vi "Config.vi"() -> ()   [LabVIEW 2020]
uses:
  Global_Variable/Global.vi
  Global_Variable/A180648.vi
  <vilib>/Utility/config.llb/NI_LVConfig.lvlib
  Libraries/S7/S7.lvlib
panel:
  in  "试验项目":T1
  in  "产品型号":string(combo)
  in  "删除":bool
  in  "确定":bool
  in  "添加":bool
  in  "退出":bool
  in  "更新":bool
  in  "选项卡控件":enum32{"产品参数", "通信参数", "系统参数"}(tab)
  in  "产品参数选项卡":T2(tab)
  in  "输入轴花键参数":string[][](table)=[[""], ["°/s"], ["°"], ["Nm"]]
  in  "输入轴移载参数":string[][](table)=[["mm"], ["mm/s"], ["mm"], ["mm/s"]]
  in  "工装参数":string[][](table)=[["mm"], ["mm/s"]]
  in  "空载判定参数":string[][](table)=[["Nm", "", ""], ["Nm", "", ""], ["Nm", "", ""], ["Nm", "", ""], ["Nm", "", ""], ["Nm", "", ""], ["Nm", "", ""], ["Nm", "", ""], ["Nm", "", ""], ["Nm", "", ""]]
  in  "空载试验参数":string[][](table)=[[""], ["°/s"], ["°"], ["Nm"]]
  in  "功能判定参数":string[][](table)=[["Nm"], ["Nm"], ["Nm"], ["Nm"], ["Nm"], ["Nm"], ["Nm"], ["Nm"], ["Nm"]]
  in  "功能试验参数":string[][](table)=[["°/s"], ["°"], ["Nm"], ["Nm"]]
  in  "车速选项卡":T3(tab)
  in  "力特性试验参数":string[][](table)=[["°/s"], ["Nm"], ["RPM"], ["Km/h"]]
  in  "传感器特性判定参数":string[][](table)=[["V", "", ""], ["V", "", ""], ["V", "", ""], ["V", "", ""], ["V", "", ""], ["V", "", ""], ["V", "", ""], ["V", "", ""], ["V", "", ""], ["V", "", ""], ["V", "", ""], ["V", "", ""], ["V", "", ""], ["V", "", ""]]
  in  "力特性判定参数 0":string[][](table)=[["Nm", "", ""], ["%", "", ""], ["Nm", "", ""], ["Nm", "", ""], ["Nm", "", ""], ["Nm", "", ""], ["Nm", "", ""], ["Nm", "", ""], ["Nm", "", ""], ["Nm", "", ""], ["Nm", "", ""], ["Nm", "", ""], ["Nm", "", ""], ["Nm", "", ""], ["Nm", "", ""], ["Nm", "", ""], ["Nm", "", ""], ["Nm", "", ""], ["Nm", "", ""], ["Nm", "", ""], ["Nm", "", ""], ["Nm", "", ""], ["Nm", "", ""], ["Nm", "", ""], ["Nm", "", ""], ["Nm", "", ""], ["Nm", "", ""]]
  in  "电流特性判定参数 0":string[][](table)=[["Nm", "", ""], ["%", "", ""], ["A", "", ""], ["A", "", ""], ["Nm", "", ""], ["Nm", "", ""], ["Nm", "", ""], ["Nm", "", ""], ["Nm", "", ""], ["Nm", "", ""], ["Nm", "", ""], ["Nm", "", ""], ["Nm", "", ""], ["Nm", "", ""], ["Nm", "", ""], ["Nm", "", ""], ["Nm", "", ""], ["Nm", "", ""], ["Nm", "", ""], ["Nm", "", ""], ["Nm", "", ""], ["Nm", "", ""], ["Nm", "", ""], ["Nm", "", ""], ["Nm", "", ""], ["Nm", "", ""], ["Nm", "", ""], ["Nm", "", ""]]
  in  "电流特性判定参数 1":string[][](table)=[["Nm", "", ""], ["%", "", ""], ["A", "", ""], ["A", "", ""], ["Nm", "", ""], ["Nm", "", ""], ["Nm", "", ""], ["Nm", "", ""], ["Nm", "", ""], ["Nm", "", ""], ["Nm", "", ""], ["Nm", "", ""], ["Nm", "", ""], ["Nm", "", ""], ["Nm", "", ""], ["Nm", "", ""], ["Nm", "", ""], ["Nm", "", ""], ["Nm", "", ""], ["Nm", "", ""], ["Nm", "", ""], ["Nm", "", ""], ["Nm", "", ""], ["Nm", "", ""], ["Nm", "", ""], ["Nm", "", ""], ["Nm", "", ""], ["Nm", "", ""]]
  in  "力特性判定参数 1":string[][](table)=[["Nm", "", ""], ["%", "", ""], ["Nm", "", ""], ["Nm", "", ""], ["Nm", "", ""], ["Nm", "", ""], ["Nm", "", ""], ["Nm", "", ""], ["Nm", "", ""], ["Nm", "", ""], ["Nm", "", ""], ["Nm", "", ""], ["Nm", "", ""], ["Nm", "", ""], ["Nm", "", ""], ["Nm", "", ""], ["Nm", "", ""], ["Nm", "", ""], ["Nm", "", ""], ["Nm", "", ""], ["Nm", "", ""], ["Nm", "", ""], ["Nm", "", ""], ["Nm", "", ""], ["Nm", "", ""], ["Nm", "", ""], ["Nm", "", ""]]
  in  "力特性判定参数 2":string[][](table)=[["Nm", "", ""], ["%", "", ""], ["Nm", "", ""], ["Nm", "", ""], ["Nm", "", ""], ["Nm", "", ""], ["Nm", "", ""], ["Nm", "", ""], ["Nm", "", ""], ["Nm", "", ""], ["Nm", "", ""], ["Nm", "", ""], ["Nm", "", ""], ["Nm", "", ""], ["Nm", "", ""], ["Nm", "", ""], ["Nm", "", ""], ["Nm", "", ""], ["Nm", "", ""], ["Nm", "", ""], ["Nm", "", ""], ["Nm", "", ""], ["Nm", "", ""], ["Nm", "", ""], ["Nm", "", ""], ["Nm", "", ""], ["Nm", "", ""]]
  in  "电流特性判定参数 2":string[][](table)=[["Nm", "", ""], ["%", "", ""], ["A", "", ""], ["A", "", ""], ["Nm", "", ""], ["Nm", "", ""], ["Nm", "", ""], ["Nm", "", ""], ["Nm", "", ""], ["Nm", "", ""], ["Nm", "", ""], ["Nm", "", ""], ["Nm", "", ""], ["Nm", "", ""], ["Nm", "", ""], ["Nm", "", ""], ["Nm", "", ""], ["Nm", "", ""], ["Nm", "", ""], ["Nm", "", ""], ["Nm", "", ""], ["Nm", "", ""], ["Nm", "", ""], ["Nm", "", ""], ["Nm", "", ""], ["Nm", "", ""], ["Nm", "", ""], ["Nm", "", ""]]
  in  "力特性判定参数 3":string[][](table)=[["Nm", "", ""], ["%", "", ""], ["Nm", "", ""], ["Nm", "", ""], ["Nm", "", ""], ["Nm", "", ""], ["Nm", "", ""], ["Nm", "", ""], ["Nm", "", ""], ["Nm", "", ""], ["Nm", "", ""], ["Nm", "", ""], ["Nm", "", ""], ["Nm", "", ""], ["Nm", "", ""], ["Nm", "", ""], ["Nm", "", ""], ["Nm", "", ""], ["Nm", "", ""], ["Nm", "", ""], ["Nm", "", ""], ["Nm", "", ""], ["Nm", "", ""], ["Nm", "", ""], ["Nm", "", ""], ["Nm", "", ""], ["Nm", "", ""]]
  in  "电流特性判定参数 3":string[][](table)=[["Nm", "", ""], ["%", "", ""], ["A", "", ""], ["A", "", ""], ["Nm", "", ""], ["Nm", "", ""], ["Nm", "", ""], ["Nm", "", ""], ["Nm", "", ""], ["Nm", "", ""], ["Nm", "", ""], ["Nm", "", ""], ["Nm", "", ""], ["Nm", "", ""], ["Nm", "", ""], ["Nm", "", ""], ["Nm", "", ""], ["Nm", "", ""], ["Nm", "", ""], ["Nm", "", ""], ["Nm", "", ""], ["Nm", "", ""], ["Nm", "", ""], ["Nm", "", ""], ["Nm", "", ""], ["Nm", "", ""], ["Nm", "", ""], ["Nm", "", ""]]
  in  "电流特性判定参数 4":string[][](table)=[["Nm", "", ""], ["%", "", ""], ["A", "", ""], ["A", "", ""], ["Nm", "", ""], ["Nm", "", ""], ["Nm", "", ""], ["Nm", "", ""], ["Nm", "", ""], ["Nm", "", ""], ["Nm", "", ""], ["Nm", "", ""], ["Nm", "", ""], ["Nm", "", ""], ["Nm", "", ""], ["Nm", "", ""], ["Nm", "", ""], ["Nm", "", ""], ["Nm", "", ""], ["Nm", "", ""], ["Nm", "", ""], ["Nm", "", ""], ["Nm", "", ""], ["Nm", "", ""], ["Nm", "", ""], ["Nm", "", ""], ["Nm", "", ""], ["Nm", "", ""]]
  in  "力特性判定参数 4":string[][](table)=[["Nm", "", ""], ["%", "", ""], ["Nm", "", ""], ["Nm", "", ""], ["Nm", "", ""], ["Nm", "", ""], ["Nm", "", ""], ["Nm", "", ""], ["Nm", "", ""], ["Nm", "", ""], ["Nm", "", ""], ["Nm", "", ""], ["Nm", "", ""], ["Nm", "", ""], ["Nm", "", ""], ["Nm", "", ""], ["Nm", "", ""], ["Nm", "", ""], ["Nm", "", ""], ["Nm", "", ""], ["Nm", "", ""], ["Nm", "", ""], ["Nm", "", ""], ["Nm", "", ""], ["Nm", "", ""], ["Nm", "", ""], ["Nm", "", ""]]
  in  "力特性判定参数 5":string[][](table)=[["Nm", "", ""], ["%", "", ""], ["Nm", "", ""], ["Nm", "", ""], ["Nm", "", ""], ["Nm", "", ""], ["Nm", "", ""], ["Nm", "", ""], ["Nm", "", ""], ["Nm", "", ""], ["Nm", "", ""], ["Nm", "", ""], ["Nm", "", ""], ["Nm", "", ""], ["Nm", "", ""], ["Nm", "", ""], ["Nm", "", ""], ["Nm", "", ""], ["Nm", "", ""], ["Nm", "", ""], ["Nm", "", ""], ["Nm", "", ""], ["Nm", "", ""], ["Nm", "", ""], ["Nm", "", ""], ["Nm", "", ""], ["Nm", "", ""]]
  in  "电流特性判定参数 5":string[][](table)=[["Nm", "", ""], ["%", "", ""], ["A", "", ""], ["A", "", ""], ["Nm", "", ""], ["Nm", "", ""], ["Nm", "", ""], ["Nm", "", ""], ["Nm", "", ""], ["Nm", "", ""], ["Nm", "", ""], ["Nm", "", ""], ["Nm", "", ""], ["Nm", "", ""], ["Nm", "", ""], ["Nm", "", ""], ["Nm", "", ""], ["Nm", "", ""], ["Nm", "", ""], ["Nm", "", ""], ["Nm", "", ""], ["Nm", "", ""], ["Nm", "", ""], ["Nm", "", ""], ["Nm", "", ""], ["Nm", "", ""], ["Nm", "", ""], ["Nm", "", ""]]
  in  "磨合参数":string[][](table)=[[""], ["°/S"], ["°"], ["Nm"]]
  in  "逆向空载判定参数":string[][](table)=[["°"], ["Nm"], ["Nm"], ["Nm"], ["Nm"], ["Nm"], ["Nm"], ["Nm"], ["Nm"], ["Nm"], ["°"], ["Nm"]]
  in  "逆向空载试验参数":string[][](table)=[[""], ["°/S"], ["°"], ["Nm"]]
  in  "振动NVH判定参数":string[][](table)
  in  "振动NVH试验参数":string[][](table)=[[""], [""], ["s"], ["s"]]
  in  "选项卡控件 2":enum32{"CAN", "K-Line"}(tab)
  in  "客户软件版本号":string
  in  "CAN_CYCLE":T4(array[cluster]) {"周期(ms)" min=1 format="%d ms"; "ID" format="0x%x"}
  in  "CAN Info":T5={"波特率"=11, "ID"=0, "帧类型"=enum."标准帧", "帧格式"=enum."数据帧", "周期(ms)"=10} caption="CAR_SPEED" {"周期(ms)" min=1 format="%d ms"; "ID" format="0x%x"; "波特率" items=["5Kbps", "10Kbps", "20Kbps", "40Kbps", "50Kbps", "80Kbps", "100Kbps", "125Kbps", "200Kbps", "250Kbps", "400Kbps", "500Kbps", "666Kbps", "800Kbps", "1000Kbps"]}
  in  "启用CAN":bool
  in  "波特率":u32=9600
  in  "诊断指令":string[][](table)
  in  "VISA resource name":refnum<visa-resource-name> caption="COM"
  in  "启用K-line诊断":bool
  in  "系统参数设置":string[][](table)
  # "性能试验台"
  # "CAN_CYCLE"
  # "帧ID"
  # "帧类型"
  # "帧格式"
  # "帧数据"
  # "周期"
types:
  T1 = cluster{"空载":bool, "功能":bool, "力特性":bool, "电流特性":bool, "传感器特性":bool, "逆向空载":bool, "振动NVH":bool, "磨合":bool}
  T2 = enum32{"输入轴", "工装", "空载", "功能", "力特性/传感器特性/电流特性/", "逆向空载/磨合", "振动NVH"}
  T3 = enum32{"设定", "车速0", "车速1", "车速2", "车速3", "车速4", "车速5"}
  T4 = cluster{"ID":u32, "帧类型":enum8{"标准帧", "扩展帧"}, "帧格式":enum16{"数据帧", "远程帧"}, "帧数据":string, "周期(ms)":u32}[]
  T5 = cluster{"波特率":u32, "ID":u32, "帧类型":enum8{"标准帧", "扩展帧"}, "帧格式":enum16{"数据帧", "远程帧"}, "周期(ms)":u32}
  T6 = enum8{"Enabled", "Disabled", "Disabled and Grayed Out"}
  T7 = typedef "NI_LVConfig.lvlib/Config Data RefNum.ctl" = refnum<k1>
  T8 = cluster{"[0]":dbl, "[1]":dbl, "[2]":dbl, "[3]":dbl}
  T9 = cluster{"[0]":cluster{string, dbl, dbl}, "[1]":cluster{string, dbl, dbl}, "[2]":cluster{string, dbl, dbl}, "[3]":cluster{string, dbl, dbl}, "[4]":cluster{string, dbl, dbl}, "[5]":cluster{string, dbl, dbl}, "[6]":cluster{string, dbl, dbl}, "[7]":cluster{string, dbl, dbl}, "[8]":cluster{string, dbl, dbl}, "[9]":cluster{string, dbl, dbl}, "[10]":cluster{string, dbl, dbl}}
  T10 = cluster{"[0]":cluster{string, dbl, dbl}, "[1]":cluster{string, dbl, dbl}, "[2]":cluster{string, dbl, dbl}, "[3]":cluster{string, dbl, dbl}, "[4]":cluster{string, dbl, dbl}, "[5]":cluster{string, dbl, dbl}, "[6]":cluster{string, dbl, dbl}, "[7]":cluster{string, dbl, dbl}, "[8]":cluster{string, dbl, dbl}, "[9]":cluster{string, dbl, dbl}}
  T11 = cluster{"[0]":cluster{string, dbl, dbl}, "[1]":cluster{string, dbl, dbl}, "[2]":cluster{string, dbl, dbl}, "[3]":cluster{string, dbl, dbl}, "[4]":cluster{string, dbl, dbl}, "[5]":cluster{string, dbl, dbl}, "[6]":cluster{string, dbl, dbl}, "[7]":cluster{string, dbl, dbl}, "[8]":cluster{string, dbl, dbl}, "[9]":cluster{string, dbl, dbl}, "[10]":cluster{string, dbl, dbl}, "[11]":cluster{string, dbl, dbl}, "[12]":cluster{string, dbl, dbl}, "[13]":cluster{string, dbl, dbl}, "[14]":cluster{string, dbl, dbl}, "[15]":cluster{string, dbl, dbl}, "[16]":cluster{string, dbl, dbl}, "[17]":cluster{string, dbl, dbl}, "[18]":cluster{string, dbl, dbl}, "[19]":cluster{string, dbl, dbl}, "[20]":cluster{string, dbl, dbl}, "[21]":cluster{string, dbl, dbl}, "[22]":cluster{string, dbl, dbl}, "[23]":cluster{string, dbl, dbl}, "[24]":cluster{string, dbl, dbl}, "[25]":cluster{string, dbl, dbl}, "[26]":cluster{string, dbl, dbl}}
  T12 = cluster{"[0]":cluster{string, dbl, dbl}, "[1]":cluster{string, dbl, dbl}, "[2]":cluster{string, dbl, dbl}, "[3]":cluster{string, dbl, dbl}, "[4]":cluster{string, dbl, dbl}, "[5]":cluster{string, dbl, dbl}, "[6]":cluster{string, dbl, dbl}, "[7]":cluster{string, dbl, dbl}, "[8]":cluster{string, dbl, dbl}, "[9]":cluster{string, dbl, dbl}, "[10]":cluster{string, dbl, dbl}, "[11]":cluster{string, dbl, dbl}, "[12]":cluster{string, dbl, dbl}, "[13]":cluster{string, dbl, dbl}}
  T13 = cluster{"[0]":cluster{string, dbl, dbl}, "[1]":cluster{string, dbl, dbl}, "[2]":cluster{string, dbl, dbl}, "[3]":cluster{string, dbl, dbl}, "[4]":cluster{string, dbl, dbl}, "[5]":cluster{string, dbl, dbl}, "[6]":cluster{string, dbl, dbl}, "[7]":cluster{string, dbl, dbl}, "[8]":cluster{string, dbl, dbl}, "[9]":cluster{string, dbl, dbl}, "[10]":cluster{string, dbl, dbl}, "[11]":cluster{string, dbl, dbl}, "[12]":cluster{string, dbl, dbl}, "[13]":cluster{string, dbl, dbl}, "[14]":cluster{string, dbl, dbl}, "[15]":cluster{string, dbl, dbl}, "[16]":cluster{string, dbl, dbl}, "[17]":cluster{string, dbl, dbl}, "[18]":cluster{string, dbl, dbl}, "[19]":cluster{string, dbl, dbl}, "[20]":cluster{string, dbl, dbl}, "[21]":cluster{string, dbl, dbl}, "[22]":cluster{string, dbl, dbl}, "[23]":cluster{string, dbl, dbl}, "[24]":cluster{string, dbl, dbl}, "[25]":cluster{string, dbl, dbl}, "[26]":cluster{string, dbl, dbl}, "[27]":cluster{string, dbl, dbl}}
  T14 = cluster{"[0]":cluster{string, dbl, dbl}, "[1]":cluster{string, dbl, dbl}, "[2]":cluster{string, dbl, dbl}, "[3]":cluster{string, dbl, dbl}, "[4]":cluster{string, dbl, dbl}, "[5]":cluster{string, dbl, dbl}, "[6]":cluster{string, dbl, dbl}, "[7]":cluster{string, dbl, dbl}, "[8]":cluster{string, dbl, dbl}, "[9]":cluster{string, dbl, dbl}, "[10]":cluster{string, dbl, dbl}, "[11]":cluster{string, dbl, dbl}}
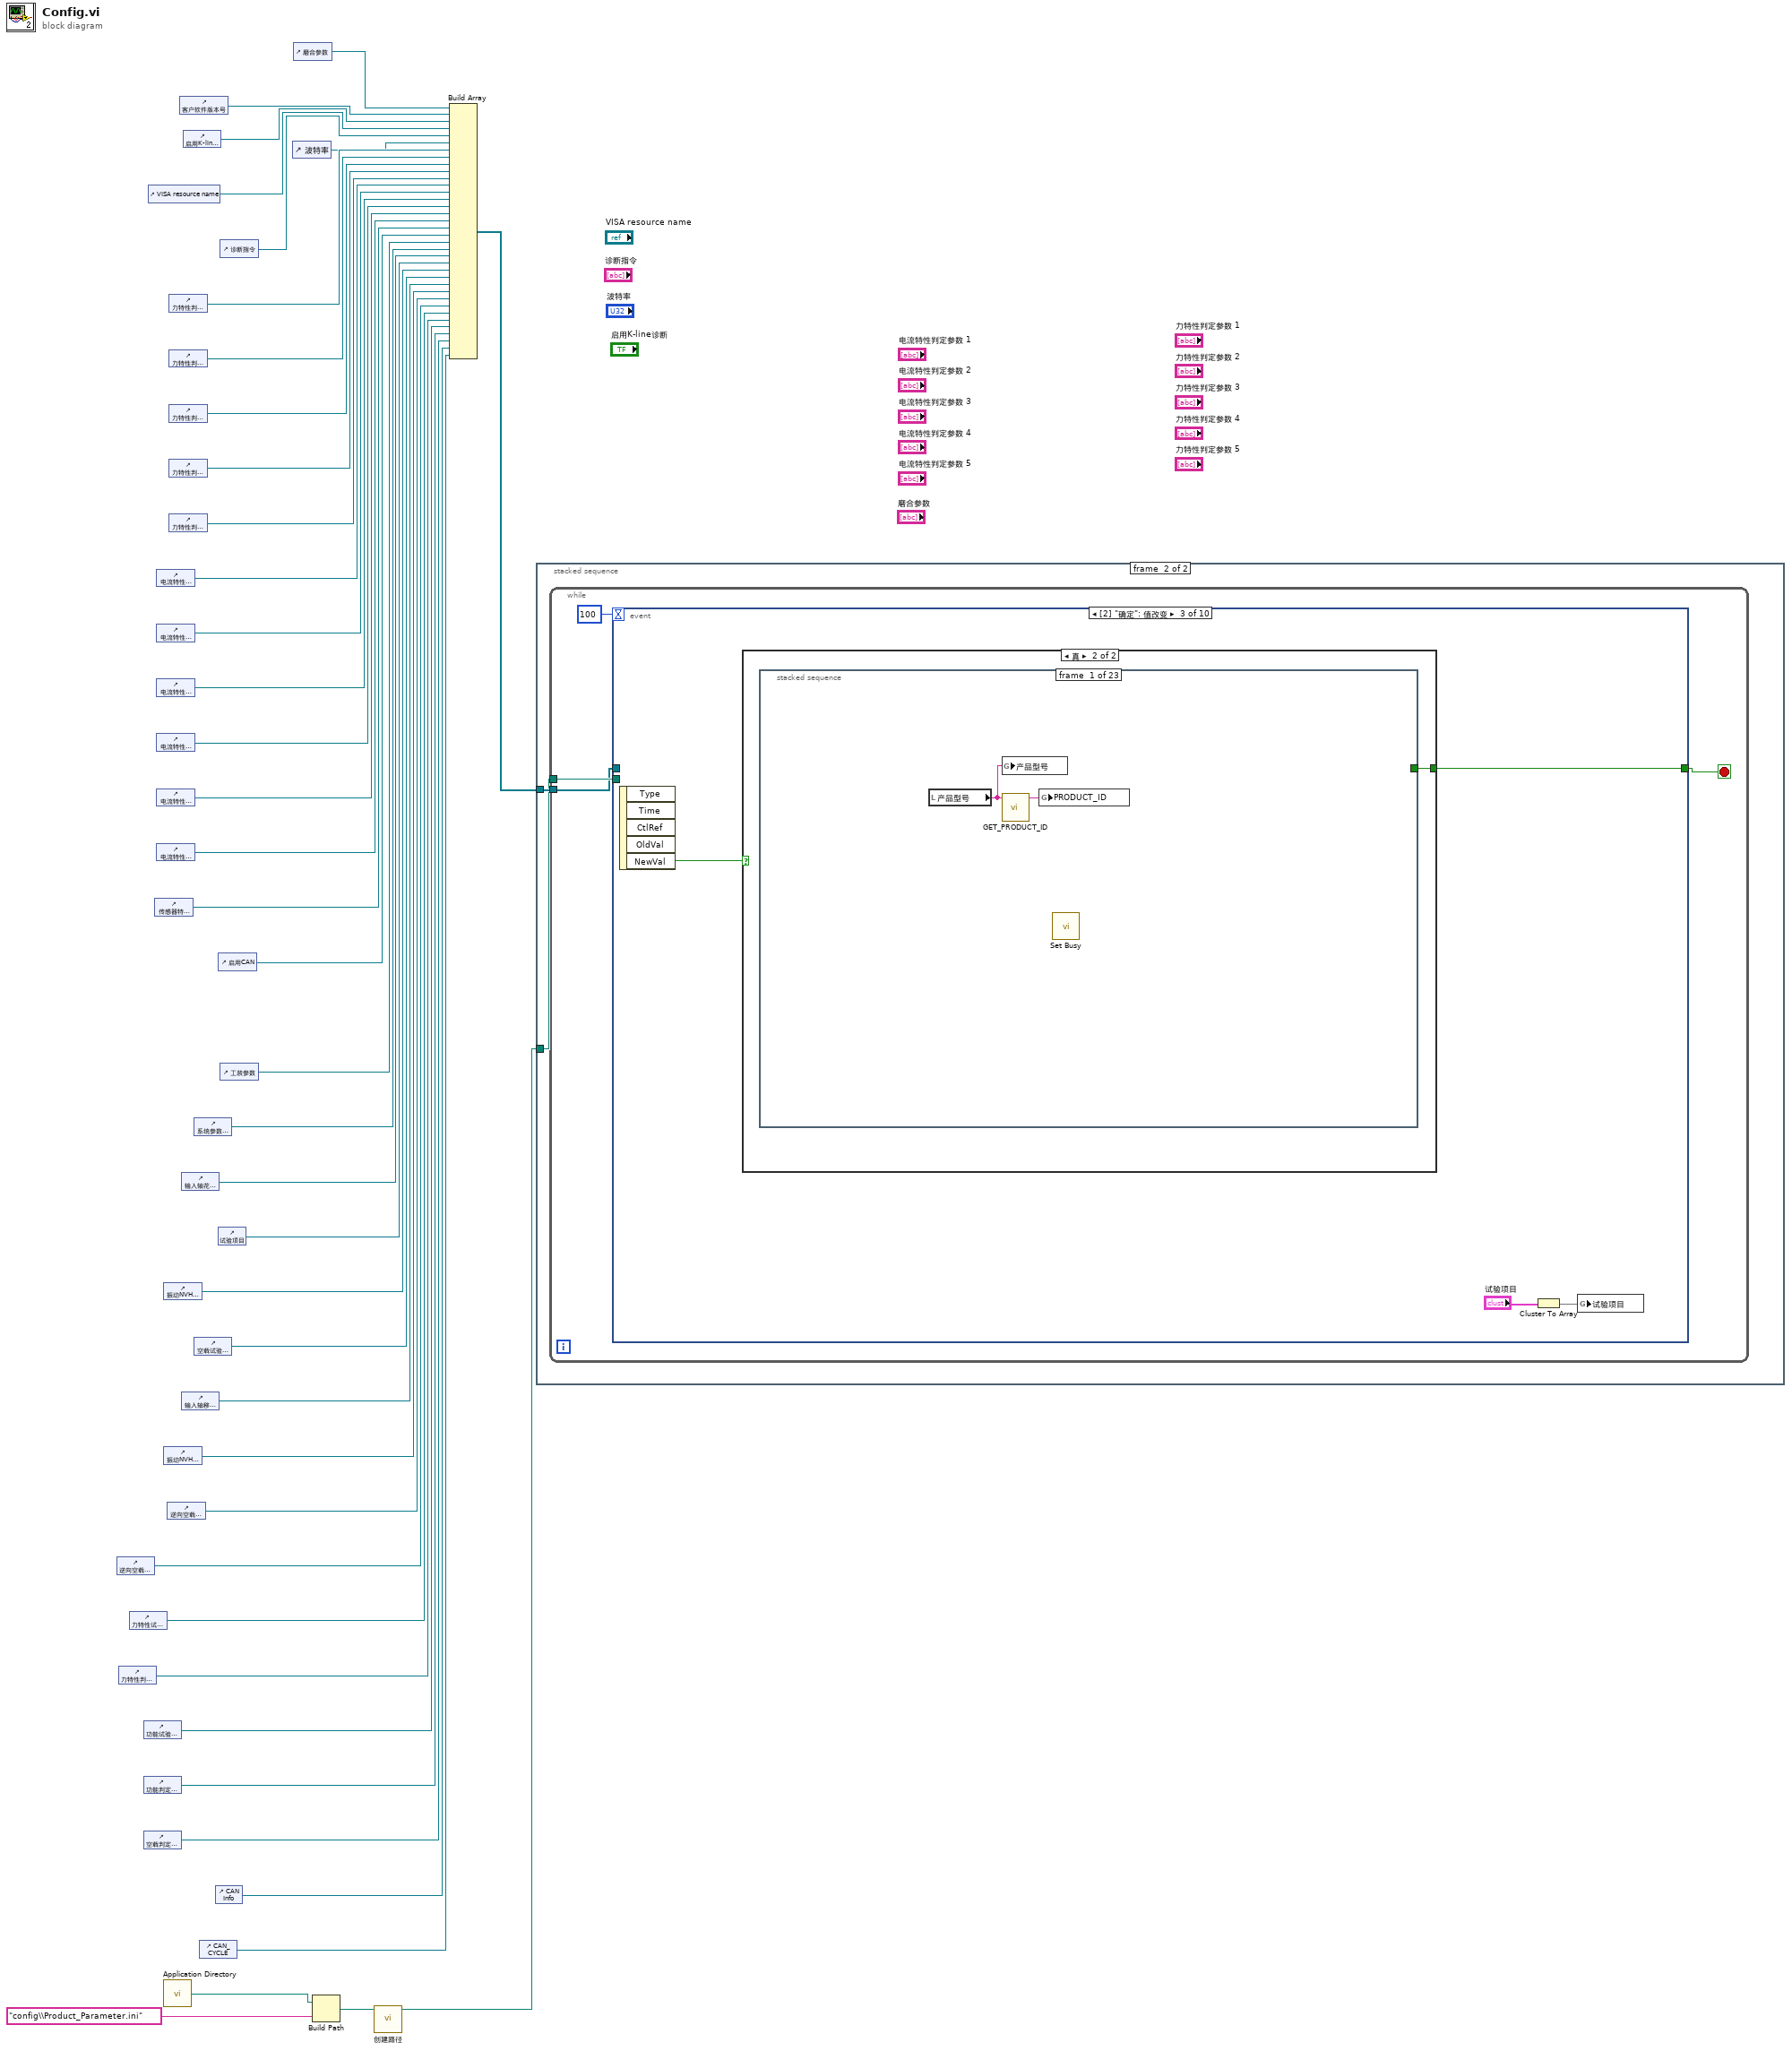
[diagram p0: block diagram]
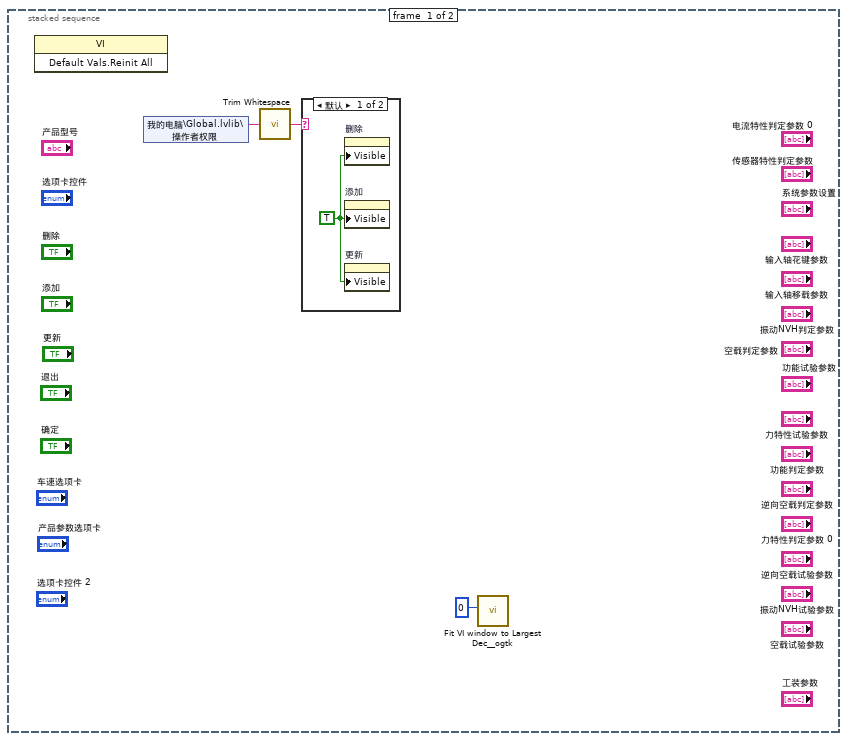
[diagram p2: hidden frame]
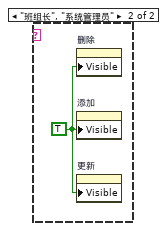
[diagram p3: hidden frame]
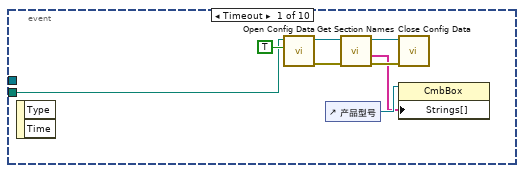
[diagram p4: hidden frame]
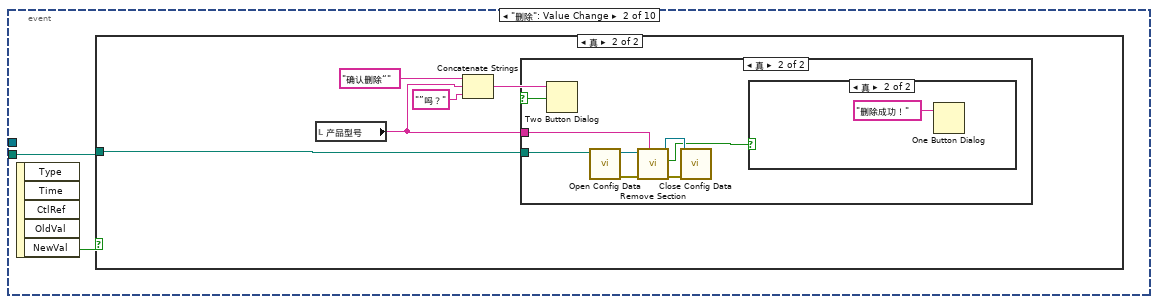
[diagram p5: hidden frame]
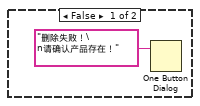
[diagram p8: hidden frame]
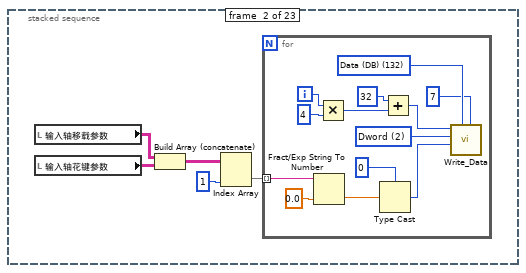
[diagram p10: hidden frame]
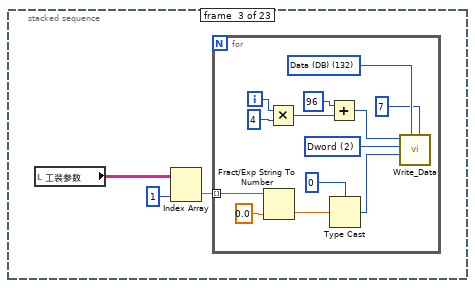
[diagram p11: hidden frame]
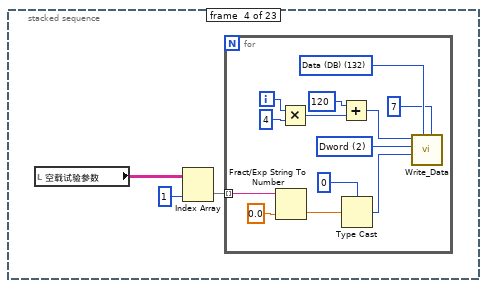
[diagram p12: hidden frame]
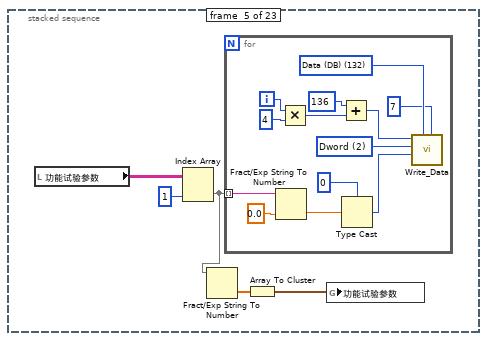
[diagram p13: hidden frame]
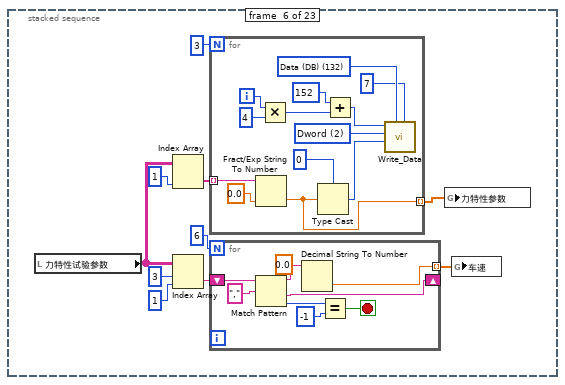
[diagram p14: hidden frame]
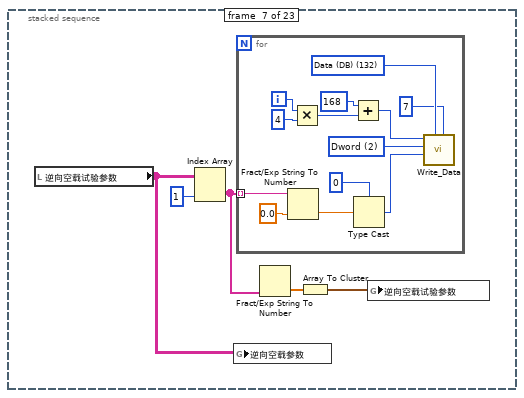
[diagram p15: hidden frame]
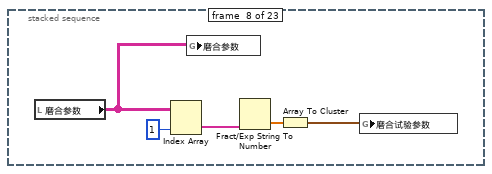
[diagram p16: hidden frame]
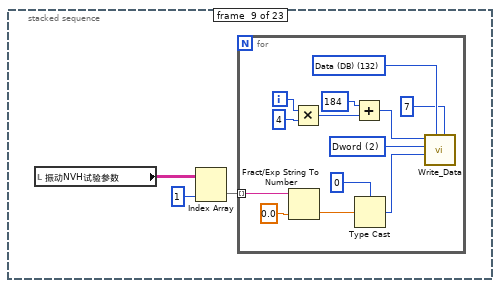
[diagram p17: hidden frame]
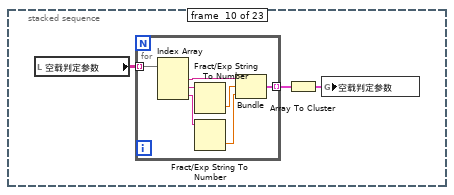
[diagram p18: hidden frame]
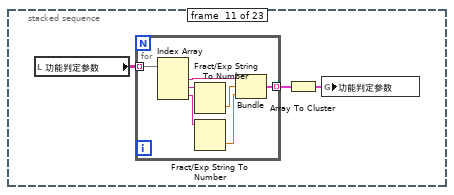
[diagram p19: hidden frame]
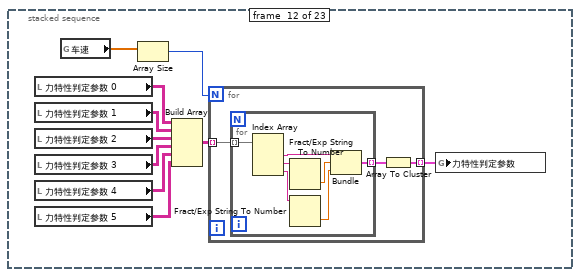
[diagram p20: hidden frame]
diagram:
  n1 = control-ref of="逆向空载判定参数"() -> (w33:refnum<vi>)
  n2 = control-ref of="力特性判定参数 0"() -> (w31:refnum<vi>)
  n3 = control-ref of="力特性试验参数"() -> (w32:refnum<vi>)
  n4 = control-ref of="功能试验参数"() -> (w30:refnum<vi>)
  n5 = control-ref of="功能判定参数"() -> (w29:refnum<vi>)
  n6 = control-ref of="空载判定参数"() -> (w28:refnum<vi>)
  n7 = control-ref of="VISA resource name"() -> (w7:refnum<vi>)
  n8 = control-ref of="传感器特性判定参数"() -> (w22:refnum<vi>)
  n9 = control-ref of="电流特性判定参数 4"() -> (w12:refnum<vi>)
  n10 = control-ref of="电流特性判定参数 3"() -> (w11:refnum<vi>)
  n11 = control-ref of="电流特性判定参数 5"() -> (w18:refnum<vi>)
  n12 = control-ref of="电流特性判定参数 2"() -> (w19:refnum<vi>)
  n13 = control-ref of="电流特性判定参数 1"() -> (w20:refnum<vi>)
  n14 = control-ref of="电流特性判定参数 0"() -> (w23:refnum<vi>)
  n15 = control-ref of="振动NVH试验参数"() -> (w38:refnum<vi>)
  n16 = control-ref of="振动NVH判定参数"() -> (w35:refnum<vi>)
  n17 = call <vilib>:"Application Directory.vi"() -> ("Application Directory"=w40:path)
  n18 = control-ref of="逆向空载试验参数"() -> (w34:refnum<vi>)
  n19 = control-ref of="力特性判定参数 3"() -> (w17:refnum<vi>)
  n20 = control-ref of="力特性判定参数 5"() -> (w16:refnum<vi>)
  n21 = control-ref of="力特性判定参数 1"() -> (w15:refnum<vi>)
  n22 = control-ref of="力特性判定参数 4"() -> (w14:refnum<vi>)
  n23 = control-ref of="力特性判定参数 2"() -> (w13:refnum<vi>)
  n24 = control-ref of="客户软件版本号"() -> (w2:refnum<vi>)
  n25 = control-ref of="输入轴花键参数"() -> (w27:refnum<vi>)
  n26 = control-ref of="输入轴移载参数"() -> (w36:refnum<vi>)
  n27 = control-ref of="启用K-line诊断"() -> (w8:refnum<vi>)
  n28 = control-ref of="系统参数设置"() -> (w26:refnum<vi>)
  n29 = control-ref of="空载试验参数"() -> (w37:refnum<vi>)
  n30 = control-ref of="CAN_CYCLE"() -> (w9:refnum<vi>)
  n31 = control-ref of="CAN Info"() -> (w21:refnum<vi>)
  n32 = control-ref of="启用CAN"() -> (w24:refnum<vi>)
  n33 = control-ref of="试验项目"() -> (w39:refnum<vi>)
  n34 = control-ref of="诊断指令"() -> (w6:refnum<vi>)
  n35 = control-ref of="工装参数"() -> (w25:refnum<vi>)
  n36 = control-ref of="波特率"() -> (w5:refnum<vi>)
  n37 = control-ref of="磨合参数"() -> (w1:refnum<vi>)
  n38 = Build Path(base path=w40, name or relative path="config\\Product_Parameter.ini" ("名称或相对路径")) -> (appended path=w4:path)
  n39 = call "创建路径.vi"("path"=w4) -> ("path out"=w3:path)  [unwired: 9 in, 1 out]
  n40 = Build Array(w1, w2, w8, w7, w6, w5, w17, w16, w15, w14, w13, w12, w11, w18, w19, w20, w23, w22, w24, w25, w26, w27, w39, w38, w37, w36, w35, w34, w33, w32, w31, w30, w29, w28, w21, w9) -> (w41:refnum<vi>[])
  n41 = stacked-sequence {
    tunnel: w41 -> [_ w48]
    tunnel: w3 -> [_ w47]
    frame #0 {
      n42 = invoke class="VI" method="Default Vals.Reinit All"() -> ()  [unwired: 3 in, 3 out]
      n43 = shared-variable "我的电脑\\Global.lvlib\\操作者权限"() -> (w44:string)  [unwired: 1 in, 1 out]
      n44 = call <vilib>:"Trim Whitespace.vi"("string"=w44) -> ("trimmed string"=w43:string)  [unwired: 1 in]
      n45 = case shown="默认" w43 {
        frame Default {
          w45 = TRUE ("可见")
          n46 = property on="删除" class="Bool (严格)"("Visible"=w45) -> ()  [unwired: 2 in, 2 out]
          n47 = property on="添加" class="Bool (严格)"("Visible"=w45) -> ()  [unwired: 2 in, 2 out]
          n48 = property on="更新" class="Bool (严格)"("Visible"=w45) -> ()  [unwired: 2 in, 2 out]
        }
        frame "班组长", "系统管理员" {
          w46 = TRUE ("可见")
          n49 = property on="删除" class="Bool (严格)"("Visible"=w46) -> ()  [unwired: 2 in, 2 out]
          n50 = property on="添加" class="Bool (严格)"("Visible"=w46) -> ()  [unwired: 2 in, 2 out]
          n51 = property on="更新" class="Bool (严格)"("Visible"=w46) -> ()  [unwired: 2 in, 2 out]
        }
      }
      n52 = call <userlib>:"Fit VI window to Largest Dec__ogtk.vi"("border spacing (2 px)"=0) -> ()  [unwired: 5 in, 2 out]
    }
    frame #1 {
      n53 = while {
        tunnel: w47 -> [w52]
        tunnel: w48 -> [w50]
        stop <- w51 stop-if-true
        n54 = event shown="[2] \"确定\": 值改变" {
          selector: _ -> [_ _ _ _ _ _ _ _ _ _]
          dyn-events: _ -> [_ _ _ _ _ _ _ _ _ _]
          timeout: 100 -> [_ _ _ _ _ _ _ _ _ _]
          tunnel: w52 -> [w55 w62 _ w336 w363 _ w387 _ _ _]
          tunnel: [_ _ w80 _ _ TRUE _ TRUE _ _] -> w51
          tunnel: w50 -> [_ _ _ w337 w364 _ w386 _ _ _]
          event Timeout {
            n55 = event-data() -> ()  [unwired: 1 in, 2 out]
            n56 = call <vilib>:"Open Config Data.vi"("create file if necessary (T)"=TRUE, "configuration file path"=w55) -> ("error out"=w57:errorcluster, "refnum"=w56:T7)  [unwired: 7 in, 1 out]
            n57 = control-ref of="产品型号"() -> (w54:refnum<vi>)
            n58 = call <vilib>:"Get Section Names.vi"("error in (no error)"=w57, "refnum"=w56) -> ("error out"=w59:errorcluster, "section names"=w53:string[], "refnum out"=w58:T7)  [unwired: 7 in]
            n59 = call <vilib>:"Close Config Data.vi"("error in (no error)"=w59, "refnum"=w58) -> ()  [unwired: 8 in, 2 out]
            n60 = property on="属性节点" class="CmbBox"(reference=w54, "Strings[]"=w53) -> ()  [unwired: 1 in, 2 out]
          }
          event "删除": Value Change {
            n61 = event-data() -> ("NewVal"=w61:bool)  [unwired: 1 in, 4 out]
            n62 = case shown="真" w61 {
              tunnel: w62 -> [_ w64]
              frame False {
              }
              frame True {
                n63 = local read "产品型号"() -> (w63:string)
                n64 = Concatenate Strings("确认删除“", w63, "”吗？") -> (w66:string)
                n65 = Two Button Dialog(message=w66) -> (T button?=w65:bool)  [unwired: 2 in]
                n66 = case shown="真" w65 {
                  tunnel: w64 -> [_ w70]
                  tunnel: w63 -> [_ w69]
                  frame False {
                  }
                  frame True {
                    n67 = call <vilib>:"Open Config Data.vi"("configuration file path"=w70) -> ("error out"=w72:errorcluster, "refnum"=w75:T7)  [unwired: 8 in, 1 out]
                    n68 = call <vilib>:"Remove Section.vi"("section"=w69, "error in (no error)"=w72, "refnum"=w75) -> ("error out"=w74:errorcluster, "section exists?"=w71:bool, "refnum out"=w73:T7)  [unwired: 6 in]
                    n69 = call <vilib>:"Close Config Data.vi"("error in (no error)"=w74, "refnum"=w73) -> ()  [unwired: 8 in, 2 out]
                    n70 = case shown="真" w71 {
                      frame False {
                        n71 = One Button Dialog(message="删除失败！\n请确认产品存在！" ("消息")) -> ()  [unwired: 1 in, 1 out]
                      }
                      frame True {
                        n72 = One Button Dialog(message="删除成功！" ("消息")) -> ()  [unwired: 1 in, 1 out]
                      }
                    }
                  }
                }
              }
            }
          }
          event "确定": Value Change {
            n73 = event-data() -> ("NewVal"=w81:bool)  [unwired: 1 in, 4 out]
            n74 = case shown="真" w81 {
              tunnel: [_ w82] -> w80
              frame False {
              }
              frame True {
                n75 = stacked-sequence {
                  tunnel: [_ _ _ _ _ _ _ _ _ _ _ _ _ _ _ _ _ _ _ _ _ _ TRUE] -> w82
                  frame #0 {
                    n76 = local read "产品型号"() -> (w84:string)
                    n77 = global write "Global.vi" "产品型号"(w84) -> ()
                    n78 = call "GET_PRODUCT_ID.vi"("PRODFUCT_NAME"=w84) -> ("PRODUCT_ID"=w83:string)  [unwired: 10 in]
                    n79 = global write "追溯Global.vi" "PRODUCT_ID"(w83) -> ()
                    n80 = call <vilib>:"Set Busy.vi"() -> ()  [unwired: 10 in, 2 out]
                  }
                  frame #1 {
                    n81 = local read "输入轴移载参数"() -> (w87:string[][])
                    n82 = local read "输入轴花键参数"() -> (w86:string[][])
                    n83 = Build Array (concatenate)(w87, w86) -> (w85:string[][])
                    n84 = Index Array(array=w85, index (col)=1 ("禁用的索引 (列)")) -> (element=w89:string[])  [unwired: 1 in]
                    n85 = for {
                      tunnel: w89 -> [w98] mode=indexing
                      i -> [w92]
                      w100 = u16 2 items=["byte", "word", "Dword"] ("数据类型")
                      w102 = u8 132 items=["I/O (P)"=128, "Input (I)"=129, "Output (Q)"=130, "Bit Memory (M)"=131, "Data (DB)"=132, "Instance Data (DI)"=133, "Local Data (L)"=134, "Predecessor Local Data (VL)"=135] ("寄存器类型")
                      n86 = Fract/Exp String To Number(string=w98, default (0 dbl)=sgl 0.0) -> (number=w96:sgl)  [unwired: 2 in, 1 out]
                      n87 = Multiply(x=w92, y=4) -> (x*y=w93:i32)
                      n88 = Type Cast(type=u32 0 ("写入地址"), x=w96) -> (*(type *) &x=w95:u32)
                      n89 = Add(x=u32 32 ("写入地址"), y=w93) -> (x+y=w90:u32)
                      n90 = call "Write_Data.vi"("DB #"=u16 7, "寄存器类型"=w102, "写入数据"=w95, "数据类型"=w100, "写入地址"=w90) -> ()  [unwired: 4 in, 3 out]
                    }
                  }
                  frame #2 {
                    n91 = local read "工装参数"() -> (w105:string[][])
                    n92 = Index Array(array=w105, index (col)=1 ("禁用的索引 (列)")) -> (element=w104:string[])  [unwired: 1 in]
                    n93 = for {
                      tunnel: w104 -> [w114] mode=indexing
                      i -> [w108]
                      w116 = u16 2 items=["byte", "word", "Dword"] ("数据类型")
                      w118 = u8 132 items=["I/O (P)"=128, "Input (I)"=129, "Output (Q)"=130, "Bit Memory (M)"=131, "Data (DB)"=132, "Instance Data (DI)"=133, "Local Data (L)"=134, "Predecessor Local Data (VL)"=135] ("寄存器类型")
                      n94 = Fract/Exp String To Number(string=w114, default (0 dbl)=sgl 0.0) -> (number=w112:sgl)  [unwired: 2 in, 1 out]
                      n95 = Multiply(x=w108, y=4) -> (x*y=w109:i32)
                      n96 = Add(x=u32 96 ("写入地址"), y=w109) -> (x+y=w106:u32)
                      n97 = Type Cast(type=u32 0 ("写入地址"), x=w112) -> (*(type *) &x=w111:u32)
                      n98 = call "Write_Data.vi"("DB #"=u16 7, "寄存器类型"=w118, "写入数据"=w111, "数据类型"=w116, "写入地址"=w106) -> ()  [unwired: 4 in, 3 out]
                    }
                  }
                  frame #3 {
                    n99 = local read "空载试验参数"() -> (w121:string[][])
                    n100 = Index Array(array=w121, index (col)=1 ("禁用的索引 (列)")) -> (element=w120:string[])  [unwired: 1 in]
                    n101 = for {
                      tunnel: w120 -> [w130] mode=indexing
                      i -> [w124]
                      w132 = u16 2 items=["byte", "word", "Dword"] ("数据类型")
                      w134 = u8 132 items=["I/O (P)"=128, "Input (I)"=129, "Output (Q)"=130, "Bit Memory (M)"=131, "Data (DB)"=132, "Instance Data (DI)"=133, "Local Data (L)"=134, "Predecessor Local Data (VL)"=135] ("寄存器类型")
                      n102 = Fract/Exp String To Number(string=w130, default (0 dbl)=sgl 0.0) -> (number=w128:sgl)  [unwired: 2 in, 1 out]
                      n103 = Multiply(x=w124, y=4) -> (x*y=w125:i32)
                      n104 = Add(x=u32 120 ("写入地址"), y=w125) -> (x+y=w122:u32)
                      n105 = Type Cast(type=u32 0 ("写入地址"), x=w128) -> (*(type *) &x=w127:u32)
                      n106 = call "Write_Data.vi"("DB #"=u16 7, "寄存器类型"=w134, "写入数据"=w127, "数据类型"=w132, "写入地址"=w122) -> ()  [unwired: 4 in, 3 out]
                    }
                  }
                  frame #4 {
                    n107 = local read "功能试验参数"() -> (w139:string[][])
                    n108 = Index Array(array=w139, index (col)=1 ("禁用的索引 (列)")) -> (element=w135:string[])  [unwired: 1 in]
                    n109 = Fract/Exp String To Number(string=w135) -> (number=w137:dbl[])  [unwired: 3 in, 1 out]
                    n110 = for {
                      tunnel: w135 -> [w148] mode=indexing
                      i -> [w142]
                      w150 = u16 2 items=["byte", "word", "Dword"] ("数据类型")
                      w152 = u8 132 items=["I/O (P)"=128, "Input (I)"=129, "Output (Q)"=130, "Bit Memory (M)"=131, "Data (DB)"=132, "Instance Data (DI)"=133, "Local Data (L)"=134, "Predecessor Local Data (VL)"=135] ("寄存器类型")
                      n111 = Fract/Exp String To Number(string=w148, default (0 dbl)=sgl 0.0) -> (number=w146:sgl)  [unwired: 2 in, 1 out]
                      n112 = Multiply(x=w142, y=4) -> (x*y=w143:i32)
                      n113 = Add(x=u32 136 ("写入地址"), y=w143) -> (x+y=w140:u32)
                      n114 = Type Cast(type=u32 0 ("写入地址"), x=w146) -> (*(type *) &x=w145:u32)
                      n115 = call "Write_Data.vi"("DB #"=u16 7, "寄存器类型"=w152, "写入数据"=w145, "数据类型"=w150, "写入地址"=w140) -> ()  [unwired: 4 in, 3 out]
                    }
                    n116 = Array To Cluster(array=w137) -> (cluster=w136:T8)
                    n117 = global write "A180648.vi" "功能试验参数"(w136) -> ()
                  }
                  frame #5 {
                    n118 = local read "力特性试验参数"() -> (w159:string[][])
                    n119 = Index Array(array=w159, index (col)=1 ("禁用的索引 (列)")) -> (element=w162:string[])  [unwired: 1 in]
                    n120 = Index Array(array=w159, index (row)=3 ("索引 (行)"), index (col)=1 ("禁用的索引 (列)")) -> (element=w156:string)
                    n121 = for {
                      N: 3 -> [_]
                      tunnel: w162 -> [w180] mode=indexing
                      tunnel: [w172] -> w153 mode=indexing
                      i -> [w175]
                      w182 = u16 2 items=["byte", "word", "Dword"] ("数据类型")
                      w184 = u8 132 items=["I/O (P)"=128, "Input (I)"=129, "Output (Q)"=130, "Bit Memory (M)"=131, "Data (DB)"=132, "Instance Data (DI)"=133, "Local Data (L)"=134, "Predecessor Local Data (VL)"=135] ("寄存器类型")
                      n122 = Fract/Exp String To Number(string=w180, default (0 dbl)=sgl 0.0) -> (number=w172:sgl)  [unwired: 2 in, 1 out]
                      n123 = Multiply(x=w175, y=4) -> (x*y=w176:i32)
                      n124 = Type Cast(type=u32 0 ("写入地址"), x=w172) -> (*(type *) &x=w178:u32)
                      n125 = Add(x=u32 152 ("写入地址"), y=w176) -> (x+y=w173:u32)
                      n126 = call "Write_Data.vi"("DB #"=u16 7, "寄存器类型"=w184, "写入数据"=w178, "数据类型"=w182, "写入地址"=w173) -> ()  [unwired: 4 in, 3 out]
                    }
                    n127 = for {
                      N: 6 -> [_]
                      shift-right: [w169] -> _
                      shift-left: w156 -> [w171]
                      tunnel: [w165] -> w155 mode=indexing
                      stop <- w164 stop-if-true
                      n128 = Match Pattern(string=w171, regular expression="," ("正则表达式")) -> (before substring=w166:string, after substring=w169:string, offset past match=w168:i32)  [unwired: 1 in, 1 out]
                      n129 = Decimal String To Number(string=w166, default (0L)=sgl 0.0 ("默认(0 I32)")) -> (number=w165:sgl)  [unwired: 1 in, 1 out]
                      n130 = Equal?(x=w168, y=-1) -> (x = y?=w164:bool)
                    }
                    n131 = global write "A180648.vi" "力特性参数"(w153) -> ()
                    n132 = global write "A180648.vi" "车速"(w155) -> ()
                  }
                  frame #6 {
                    n133 = local read "逆向空载试验参数"() -> (w185:string[][])
                    n134 = Index Array(array=w185, index (col)=1 ("禁用的索引 (列)")) -> (element=w186:string[])  [unwired: 1 in]
                    n135 = global write "A180648.vi" "逆向空载参数"(w185) -> ()
                    n136 = for {
                      tunnel: w186 -> [w198] mode=indexing
                      i -> [w192]
                      w200 = u16 2 items=["byte", "word", "Dword"] ("数据类型")
                      w202 = u8 132 items=["I/O (P)"=128, "Input (I)"=129, "Output (Q)"=130, "Bit Memory (M)"=131, "Data (DB)"=132, "Instance Data (DI)"=133, "Local Data (L)"=134, "Predecessor Local Data (VL)"=135] ("寄存器类型")
                      n137 = Fract/Exp String To Number(string=w198, default (0 dbl)=sgl 0.0) -> (number=w196:sgl)  [unwired: 2 in, 1 out]
                      n138 = Multiply(x=w192, y=4) -> (x*y=w193:i32)
                      n139 = Add(x=u32 168 ("写入地址"), y=w193) -> (x+y=w190:u32)
                      n140 = Type Cast(type=u32 0 ("写入地址"), x=w196) -> (*(type *) &x=w195:u32)
                      n141 = call "Write_Data.vi"("DB #"=u16 7, "寄存器类型"=w202, "写入数据"=w195, "数据类型"=w200, "写入地址"=w190) -> ()  [unwired: 4 in, 3 out]
                    }
                    n142 = Fract/Exp String To Number(string=w186) -> (number=w188:dbl[])  [unwired: 3 in, 1 out]
                    n143 = Array To Cluster(array=w188) -> (cluster=w187:T8)
                    n144 = global write "A180648.vi" "逆向空载试验参数"(w187) -> ()
                  }
                  frame #7 {
                    n145 = local read "磨合参数"() -> (w203:string[][])
                    n146 = Index Array(array=w203, index (col)=1 ("禁用的索引 (列)")) -> (element=w204:string[])  [unwired: 1 in]
                    n147 = global write "A180648.vi" "磨合参数"(w203) -> ()
                    n148 = Fract/Exp String To Number(string=w204) -> (number=w206:dbl[])  [unwired: 3 in, 1 out]
                    n149 = Array To Cluster(array=w206) -> (cluster=w205:T8)
                    n150 = global write "A180648.vi" "磨合试验参数"(w205) -> ()
                  }
                  frame #8 {
                    n151 = local read "振动NVH试验参数"() -> (w210:string[][])
                    n152 = Index Array(array=w210, index (col)=1 ("禁用的索引 (列)")) -> (element=w209:string[])  [unwired: 1 in]
                    n153 = for {
                      tunnel: w209 -> [w219] mode=indexing
                      i -> [w213]
                      w221 = u16 2 items=["byte", "word", "Dword"] ("数据类型")
                      w223 = u8 132 items=["I/O (P)"=128, "Input (I)"=129, "Output (Q)"=130, "Bit Memory (M)"=131, "Data (DB)"=132, "Instance Data (DI)"=133, "Local Data (L)"=134, "Predecessor Local Data (VL)"=135] ("寄存器类型")
                      n154 = Fract/Exp String To Number(string=w219, default (0 dbl)=sgl 0.0) -> (number=w217:sgl)  [unwired: 2 in, 1 out]
                      n155 = Multiply(x=w213, y=4) -> (x*y=w214:i32)
                      n156 = Add(x=u32 184 ("写入地址"), y=w214) -> (x+y=w211:u32)
                      n157 = Type Cast(type=u32 0 ("写入地址"), x=w217) -> (*(type *) &x=w216:u32)
                      n158 = call "Write_Data.vi"("DB #"=u16 7, "寄存器类型"=w223, "写入数据"=w216, "数据类型"=w221, "写入地址"=w211) -> ()  [unwired: 4 in, 3 out]
                    }
                  }
                  frame #9 {
                    n159 = local read "空载判定参数"() -> (w226:string[][])
                    n160 = for {
                      tunnel: w226 -> [w233] mode=indexing
                      tunnel: [w228] -> w225 mode=indexing
                      n161 = Index Array(array=w233) -> (element #1=w227:string, element #2=w232:string, element #3=w231:string)  [unwired: 3 in]
                      n162 = Fract/Exp String To Number(string=w232) -> (number=w230:dbl)  [unwired: 3 in, 1 out]
                      n163 = Fract/Exp String To Number(string=w231) -> (number=w229:dbl)  [unwired: 3 in, 1 out]
                      n164 = Bundle(w227, w230, w229) -> (w228:cluster{string, dbl, dbl})  [unwired: 1 in]
                    }
                    n165 = Array To Cluster(array=w225) -> (cluster=w224:T9)
                    n166 = global write "判定参数.vi" "空载判定参数"(w224) -> ()
                  }
                  frame #10 {
                    n167 = local read "功能判定参数"() -> (w236:string[][])
                    n168 = for {
                      tunnel: w236 -> [w243] mode=indexing
                      tunnel: [w238] -> w235 mode=indexing
                      n169 = Index Array(array=w243) -> (element #1=w237:string, element #2=w242:string, element #3=w241:string)  [unwired: 3 in]
                      n170 = Fract/Exp String To Number(string=w242) -> (number=w240:dbl)  [unwired: 3 in, 1 out]
                      n171 = Fract/Exp String To Number(string=w241) -> (number=w239:dbl)  [unwired: 3 in, 1 out]
                      n172 = Bundle(w237, w240, w239) -> (w238:cluster{string, dbl, dbl})  [unwired: 1 in]
                    }
                    n173 = Array To Cluster(array=w235) -> (cluster=w234:T10)
                    n174 = global write "判定参数.vi" "功能判定参数"(w234) -> ()
                  }
                  frame #11 {
                    n175 = local read "力特性判定参数 0"() -> (w253:string[][])
                    n176 = local read "力特性判定参数 1"() -> (w252:string[][])
                    n177 = local read "力特性判定参数 2"() -> (w251:string[][])
                    n178 = local read "力特性判定参数 3"() -> (w250:string[][])
                    n179 = local read "力特性判定参数 4"() -> (w249:string[][])
                    n180 = local read "力特性判定参数 5"() -> (w248:string[][])
                    n181 = global read "A180648.vi" "车速"() -> (w245:sgl[])
                    n182 = Array Size(array=w245) -> (size(s)=w244:i32)
                    n183 = Build Array(w253, w252, w251, w250, w249, w248) -> (w247:string[][][])
                    n184 = for {
                      N: w244 -> [_]
                      tunnel: [w255] -> w246 mode=indexing
                      tunnel: w247 -> [w256] mode=indexing
                      n185 = for {
                        tunnel: w256 -> [w263] mode=indexing
                        tunnel: [w257] -> w254 mode=indexing
                        n186 = Index Array(array=w263) -> (element #1=w258:string, element #2=w262:string, element #3=w261:string)  [unwired: 3 in]
                        n187 = Fract/Exp String To Number(string=w262) -> (number=w260:dbl)  [unwired: 3 in, 1 out]
                        n188 = Fract/Exp String To Number(string=w261) -> (number=w259:dbl)  [unwired: 3 in, 1 out]
                        n189 = Bundle(w258, w260, w259) -> (w257:cluster{string, dbl, dbl})  [unwired: 1 in]
                      }
                      n190 = Array To Cluster(array=w254) -> (cluster=w255:T11)
                    }
                    n191 = global write "判定参数.vi" "力特性判定参数"(w246) -> ()
                  }
                  frame #12 {
                    n192 = local read "传感器特性判定参数"() -> (w266:string[][])
                    n193 = for {
                      tunnel: w266 -> [w273] mode=indexing
                      tunnel: [w268] -> w265 mode=indexing
                      n194 = Index Array(array=w273) -> (element #1=w267:string, element #2=w272:string, element #3=w271:string)  [unwired: 3 in]
                      n195 = Fract/Exp String To Number(string=w272) -> (number=w270:dbl)  [unwired: 3 in, 1 out]
                      n196 = Fract/Exp String To Number(string=w271) -> (number=w269:dbl)  [unwired: 3 in, 1 out]
                      n197 = Bundle(w267, w270, w269) -> (w268:cluster{string, dbl, dbl})  [unwired: 1 in]
                    }
                    n198 = Array To Cluster(array=w265) -> (cluster=w264:T12)
                    n199 = global write "判定参数.vi" "传感器特性判定参数"(w264) -> ()
                  }
                  frame #13 {
                    n200 = local read "电流特性判定参数 0"() -> (w283:string[][])
                    n201 = local read "电流特性判定参数 1"() -> (w282:string[][])
                    n202 = local read "电流特性判定参数 2"() -> (w281:string[][])
                    n203 = local read "电流特性判定参数 3"() -> (w280:string[][])
                    n204 = local read "电流特性判定参数 4"() -> (w279:string[][])
                    n205 = local read "电流特性判定参数 5"() -> (w278:string[][])
                    n206 = global read "A180648.vi" "车速"() -> (w275:sgl[])
                    n207 = Array Size(array=w275) -> (size(s)=w274:i32)
                    n208 = Build Array(w283, w282, w281, w280, w279, w278) -> (w277:string[][][])
                    n209 = for {
                      N: w274 -> [_]
                      tunnel: [w285] -> w276 mode=indexing
                      tunnel: w277 -> [w286] mode=indexing
                      n210 = for {
                        tunnel: w286 -> [w293] mode=indexing
                        tunnel: [w287] -> w284 mode=indexing
                        n211 = Index Array(array=w293) -> (element #1=w288:string, element #2=w292:string, element #3=w291:string)  [unwired: 3 in]
                        n212 = Fract/Exp String To Number(string=w292) -> (number=w290:dbl)  [unwired: 3 in, 1 out]
                        n213 = Fract/Exp String To Number(string=w291) -> (number=w289:dbl)  [unwired: 3 in, 1 out]
                        n214 = Bundle(w288, w290, w289) -> (w287:cluster{string, dbl, dbl})  [unwired: 1 in]
                      }
                      n215 = Array To Cluster(array=w284) -> (cluster=w285:T13)
                    }
                    n216 = global write "判定参数.vi" "电流特性判定参数"(w276) -> ()
                  }
                  frame #14 {
                    n217 = local read "逆向空载判定参数"() -> (w296:string[][])
                    n218 = for {
                      tunnel: w296 -> [w303] mode=indexing
                      tunnel: [w298] -> w295 mode=indexing
                      n219 = Index Array(array=w303) -> (element #1=w297:string, element #2=w302:string, element #3=w301:string)  [unwired: 3 in]
                      n220 = Fract/Exp String To Number(string=w302) -> (number=w300:dbl)  [unwired: 3 in, 1 out]
                      n221 = Fract/Exp String To Number(string=w301) -> (number=w299:dbl)  [unwired: 3 in, 1 out]
                      n222 = Bundle(w297, w300, w299) -> (w298:cluster{string, dbl, dbl})  [unwired: 1 in]
                    }
                    n223 = Array To Cluster(array=w295) -> (cluster=w294:T14)
                    n224 = global write "判定参数.vi" "逆向空载判定参数"(w294) -> ()
                  }
                  frame #15 {
                    n225 = local read "振动NVH判定参数"() -> (w309:string[][])
                    n226 = for {
                      tunnel: w309 -> [w316] mode=indexing
                      tunnel: [w311] -> w308 mode=indexing
                      n227 = Index Array(array=w316) -> (element #1=w310:string, element #2=w315:string, element #3=w314:string)  [unwired: 3 in]
                      n228 = Fract/Exp String To Number(string=w315) -> (number=w313:dbl)  [unwired: 3 in, 1 out]
                      n229 = Fract/Exp String To Number(string=w314) -> (number=w312:dbl)  [unwired: 3 in, 1 out]
                      n230 = Bundle(w310, w313, w312) -> (w311:cluster{string, dbl, dbl})  [unwired: 1 in]
                    }
                    n231 = Decimate 1D Array(w308) -> (w307:cluster{string, dbl, dbl}[], w305:cluster{string, dbl, dbl}[])
                    n232 = Array To Cluster(array=w307) -> (cluster=w306:T10)
                    n233 = Array To Cluster(array=w305) -> (cluster=w304:T10)
                    n234 = global write "判定参数.vi" "振动判定范围"(w306) -> ()
                    n235 = global write "判定参数.vi" "振动判定"(w304) -> ()
                  }
                  frame #16 {
                    n236 = global write "Global.vi" "CAN Info"("CAN Info") -> ()
                    n237 = global write "Global.vi" "启用CAN"("启用CAN") -> ()
                    n238 = global write "Global.vi" "CAN_CYCLE"("CAN_CYCLE") -> ()
                    n239 = global write "Global.vi" "CAN软件版本号"("客户软件版本号") -> ()
                  }
                  frame #17 {
                    n240 = disable-structure shown="禁用" {
                      frame Disabled {
                        n241 = local read "系统参数设置"() -> (w325:string[][])
                        n242 = Index Array(array=w325, index (col)=0 ("禁用的索引 (列)")) -> (element=w323:string[])  [unwired: 1 in]
                        n243 = Index Array(array=w323) -> (element #1=w322:string, element #2=w321:string)  [unwired: 2 in]
                        n244 = global write "Global.vi" "软件版本号"(w322) -> ()
                        n245 = global write "Global.vi" "硬件版本号"(w321) -> ()
                      }
                      frame Enabled {
                      }
                    }
                  }
                  frame #18 {
                    n246 = local read "波特率"() -> (w329:u32)
                    n247 = local read "诊断指令"() -> (w328:string[][])
                    n248 = local read "启用K-line诊断"() -> (w326:bool)
                    n249 = local read "VISA resource name"() -> (w327:refnum<visa-resource-name>)
                    n250 = global write "Global.vi" "VISA resource name"(w327) -> ()
                    n251 = global write "Global.vi" "启用K-line诊断"(w326) -> ()
                    n252 = global write "Global.vi" "K-Line波特率"(w329) -> ()
                    n253 = global write "Global.vi" "诊断指令"(w328) -> ()
                  }
                  frame #19 {
                    n254 = call <vilib>:"Unset Busy.vi"() -> ()  [unwired: 11 in, 1 out]
                  }
                  frame #20 {
                    n255 = global read "Global.vi" "更换产品"() -> (w331:refnum<vi>)
                    n256 = vi-ref "Auto.vi"() -> (w330:refnum<vi>)
                    n257 = property class="VIRef"(reference=w331, "Val(Sgnl)"=w330) -> ()  [unwired: 1 in, 2 out]
                  }
                  frame #21 {
                    w332 = "参数装载成功！" ("消息")
                    n258 = call "浮动通知.vi"("通知内容"=w332) -> ()  [unwired: 11 in]
                    n259 = One Button Dialog(message=w332) -> ()  [unwired: 1 in, 1 out]
                  }
                  frame #22 {
                    n260 = control-ref of="本VI"() -> (w333:refnum<vi>)
                    n261 = invoke class="VI" method="FP.Close"(reference=w333) -> ()  [unwired: 2 in, 3 out]
                  }
                }
              }
            }
            n262 = Cluster To Array(cluster="试验项目") -> (array=w78:bool[])
            n263 = global write "Global.vi" "试验项目"(w78) -> ()
          }
          event "添加": Value Change {
            n264 = event-data() -> ("NewVal"=w335:bool)  [unwired: 1 in, 4 out]
            n265 = case shown="真" w335 {
              tunnel: w337 -> [_ w341]
              tunnel: w336 -> [_ w340]
              frame False {
              }
              frame True {
                n266 = call "产品添加提示：用户输入"() -> ("产品型号"=w338:string, "确定"=w339:bool)  [unwired: 17 in, 1 out]
                n267 = case shown="真" w339 {
                  tunnel: w341 -> [_ w344]
                  tunnel: w340 -> [_ w343]
                  tunnel: w338 -> [_ w342]
                  frame False {
                  }
                  frame True {
                    n268 = case shown="默认" w342 {
                      selector: w342 -> [_ w347]
                      tunnel: w344 -> [_ w350]
                      tunnel: w343 -> [_ w349]
                      frame "" {
                        n269 = One Button Dialog(message="产品名称不得为空!" ("text")) -> ()  [unwired: 1 in, 1 out]
                      }
                      frame Default {
                        n270 = property on="产品型号" class="CmbBox"() -> ("Strings[]"=w348:string[])  [unwired: 2 in, 2 out]
                        n271 = Search 1D Array(1D array=w348, element=w347) -> (index of element=w346:i32)  [unwired: 1 in]
                        n272 = case shown="-1" w346 {
                          tunnel: w350 -> [_ w354]
                          tunnel: w349 -> [_ w353]
                          tunnel: w347 -> [_ w352]
                          frame Default {
                            n273 = One Button Dialog(message="产品已存在！" ("消息")) -> ()  [unwired: 1 in, 1 out]
                          }
                          frame -1 {
                            n274 = stacked-sequence {
                              tunnel: w354 -> [w360 _]
                              tunnel: w353 -> [w359 _]
                              tunnel: w352 -> [w358 _]
                              frame #0 {
                                n275 = call <vilib>:"Set Busy.vi"() -> ("error out"=w356:errorcluster)  [unwired: 10 in, 1 out]
                                n276 = call "Read_Write INI File.vi"("Mode"=enum16{"Read", "Write"}."Write", "Section"=w358, "error in"=w356, "Filepath"=w359, "Ctl Refnum"=w360) -> ("error out"=w355:errorcluster)  [unwired: 6 in]
                                n277 = call <vilib>:"Unset Busy.vi"("error in (no error)"=w355) -> ()  [unwired: 10 in, 1 out]
                              }
                              frame #1 {
                                n278 = One Button Dialog(message="添加成功！" ("消息")) -> ()  [unwired: 1 in, 1 out]
                              }
                            }
                          }
                        }
                      }
                    }
                  }
                }
              }
            }
          }
          event "产品型号": Value Change {
            n279 = event-data() -> ("NewVal"=w362:string)  [unwired: 1 in, 4 out]
            n280 = stacked-sequence {
              tunnel: w364 -> [_ _ w368]
              tunnel: w363 -> [_ _ w367]
              tunnel: w362 -> [_ w366 _]
              frame #0 {
                n281 = control-ref of="本VI"() -> (w365:refnum<vi>)
                n282 = invoke class="VI" method="Default Vals.Reinit All"(reference=w365) -> ()  [unwired: 2 in, 3 out]
              }
              frame #1 {
                n283 = local write "产品型号"(w366) -> ()
              }
              frame #2 {
                n284 = disable-structure shown="启用" {
                  disable-tunnel: w368 -> [w370 w379]
                  disable-tunnel: w367 -> [w369 w380]
                  frame Disabled {
                    n285 = for {
                      tunnel: w370 -> [w373] mode=indexing
                      tunnel: w369 -> [w372]
                      n286 = local read "产品型号"() -> (w371:string)
                      n287 = call "Read_Write ParaINI File.vi"("Mode"=enum16{"Read", "Write"}."Read", "Section"=w371, "Filepath"=w372, "Ctl Refnum"=w373) -> ()  [unwired: 7 in, 1 out]
                    }
                  }
                  frame Enabled {
                    n288 = call <vilib>:"Set Busy.vi"() -> ("error out"=w375:errorcluster)  [unwired: 10 in, 1 out]
                    n289 = local read "产品型号"() -> (w378:string)
                    n290 = call "Read_Write INI File.vi"("Mode"=enum16{"Read", "Write"}."Read", "Section"=w378, "error in"=w375, "Filepath"=w380, "Ctl Refnum"=w379) -> ("error out"=w376:errorcluster)  [unwired: 6 in]
                    n291 = call <vilib>:"Unset Busy.vi"("error in (no error)"=w376) -> ()  [unwired: 10 in, 1 out]
                  }
                }
              }
            }
          }
          event "退出": Value Change {
            n292 = event-data() -> ()  [unwired: 1 in, 5 out]
            n293 = control-ref of="本VI"() -> (w383:refnum<vi>)
            n294 = invoke class="VI" method="FP.Close"(reference=w383) -> (reference out=w381:refnum<vi>, error out=w382:errorcluster)  [unwired: 2 in, 1 out]
            n295 = Close Reference(reference=w381, error in (no error)=w382) -> ()  [unwired: 1 out]
          }
          event "更新": Value Change {
            n296 = event-data() -> ("NewVal"=w385:bool)  [unwired: 1 in, 4 out]
            n297 = case shown="真" w385 {
              tunnel: w387 -> [_ w390]
              tunnel: w386 -> [_ w389]
              frame False {
              }
              frame True {
                n298 = disable-structure shown="启用" {
                  disable-tunnel: w390 -> [w393 w404]
                  disable-tunnel: w389 -> [w392 w399]
                  disable-tunnel: [w391 w401] -> w388
                  frame Disabled {
                    n299 = for {
                      tunnel: w393 -> [w396]
                      tunnel: w392 -> [w395] mode=indexing
                      tunnel: [w394] -> w391
                      n300 = local read "产品型号"() -> (w398:string)
                      n301 = call "Read_Write ParaINI File.vi"("Mode"=enum16{"Read", "Write"}."Write", "Section"=w398, "Filepath"=w396, "Ctl Refnum"=w395) -> ("error out"=w394:errorcluster)  [unwired: 7 in]
                    }
                  }
                  frame Enabled {
                    n302 = call <vilib>:"Set Busy.vi"() -> ("error out"=w400:errorcluster)  [unwired: 10 in, 1 out]
                    n303 = local read "产品型号"() -> (w403:string)
                    n304 = call "Read_Write INI File.vi"("Mode"=enum16{"Read", "Write"}."Write", "Section"=w403, "error in"=w400, "Filepath"=w404, "Ctl Refnum"=w399) -> ("error out"=w401:errorcluster)  [unwired: 6 in]
                  }
                }
                n305 = case shown="无错误" w388 {
                  frame No Error {
                    n306 = call <vilib>:"Unset Busy.vi"() -> ()  [unwired: 11 in, 1 out]
                    n307 = Wait (ms)(milliseconds to wait=u32 500 ("等待时间（毫秒）")) -> ()  [unwired: 1 out]
                    n308 = One Button Dialog(message="更新成功！" ("通知内容")) -> ()  [unwired: 1 in, 1 out]
                  }
                  frame Error {
                    n309 = Wait (ms)(milliseconds to wait=u32 500 ("等待时间（毫秒）")) -> ()  [unwired: 1 out]
                    n310 = call "浮动通知.vi"("通知内容"="更新失败！") -> ()  [unwired: 11 in]
                  }
                }
              }
            }
          }
          event Panel Close {
            n311 = event-data() -> ()  [unwired: 1 in, 3 out]
          }
          event "启用CAN": Value Change {
            n312 = event-data() -> ("NewVal"=w410:bool)  [unwired: 1 in]
            n313 = case shown="真" w410 {
              frame False {
                n314 = control-ref of="CAN_CYCLE"() -> (w412:refnum<vi>)
                n315 = control-ref of="CAN Info"() -> (w413:refnum<vi>)
                n316 = Build Array(w413, w412) -> (w411:refnum<vi>[])
                n317 = for {
                  tunnel: w411 -> [w415] mode=indexing
                  n318 = property class="Ctl"(reference=w415, "DisabledEnum"=T6."Disabled and Grayed Out" ("禁用")) -> ()  [unwired: 1 in, 2 out]
                }
              }
              frame True {
                n319 = control-ref of="VISA resource name"() -> (w421:refnum<vi>)
                n320 = local write "启用K-line诊断"(FALSE ("启用K-line诊断")) -> ()
                n321 = control-ref of="CAN_CYCLE"() -> (w417:refnum<vi>)
                n322 = control-ref of="诊断指令"() -> (w422:refnum<vi>)
                n323 = control-ref of="波特率"() -> (w423:refnum<vi>)
                n324 = control-ref of="CAN Info"() -> (w418:refnum<vi>)
                n325 = Build Array(w423, w422, w421) -> (w420:refnum<vi>[])
                n326 = Build Array(w418, w417) -> (w416:refnum<vi>[])
                n327 = for {
                  tunnel: w420 -> [w427] mode=indexing
                  n328 = property class="Ctl"(reference=w427, "DisabledEnum"=T6."Disabled and Grayed Out" ("禁用")) -> ()  [unwired: 1 in, 2 out]
                }
                n329 = for {
                  tunnel: w416 -> [w425] mode=indexing
                  n330 = property class="Ctl"(reference=w425, "DisabledEnum"=T6."Enabled" ("禁用")) -> ()  [unwired: 1 in, 2 out]
                }
              }
            }
          }
          event "启用K-line诊断": Value Change {
            n331 = event-data() -> ("NewVal"=w428:bool)  [unwired: 1 in]
            n332 = case shown="假" w428 {
              frame False {
                n333 = control-ref of="VISA resource name"() -> (w430:refnum<vi>)
                n334 = control-ref of="诊断指令"() -> (w431:refnum<vi>)
                n335 = control-ref of="波特率"() -> (w432:refnum<vi>)
                n336 = Build Array(w432, w431, w430) -> (w429:refnum<vi>[])
                n337 = for {
                  tunnel: w429 -> [w434] mode=indexing
                  n338 = property class="Ctl"(reference=w434, "DisabledEnum"=T6."Enabled" ("禁用")) -> ()  [unwired: 1 in, 2 out]
                }
              }
              frame True {
                n339 = control-ref of="VISA resource name"() -> (w440:refnum<vi>)
                n340 = local write "启用CAN"(FALSE ("启用K-line诊断")) -> ()
                n341 = control-ref of="CAN_CYCLE"() -> (w436:refnum<vi>)
                n342 = control-ref of="诊断指令"() -> (w441:refnum<vi>)
                n343 = control-ref of="波特率"() -> (w442:refnum<vi>)
                n344 = control-ref of="CAN Info"() -> (w437:refnum<vi>)
                n345 = Build Array(w442, w441, w440) -> (w439:refnum<vi>[])
                n346 = Build Array(w437, w436) -> (w435:refnum<vi>[])
                n347 = for {
                  tunnel: w439 -> [w446] mode=indexing
                  n348 = property class="Ctl"(reference=w446, "DisabledEnum"=T6."Enabled" ("禁用")) -> ()  [unwired: 1 in, 2 out]
                }
                n349 = for {
                  tunnel: w435 -> [w444] mode=indexing
                  n350 = property class="Ctl"(reference=w444, "DisabledEnum"=T6."Disabled and Grayed Out" ("禁用")) -> ()  [unwired: 1 in, 2 out]
                }
              }
            }
          }
        }
      }
    }
  }
